vi "Gradient Read Array.vi"(8 "error in":errorcluster, 11 "Flow Gradient in":refnum<class "Flow Gradient.lvclass">) -> (0 "error out":errorcluster, 1 "Changed or First Call?":bool, 2 "Flow SP":dbl[](array[numeric]), 3 "Flow Gradient out":refnum<class "Flow Gradient.lvclass">)   [LabVIEW 2023, in "Flow Gradient.lvclass"]
uses:
  Flow Gradient.lvclass
  Parents/Gradient/Gradient.lvclass
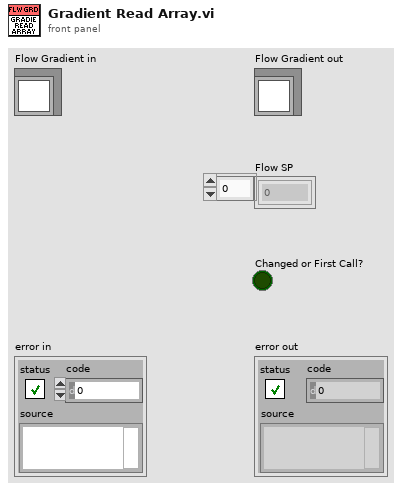
[diagram p1: front panel]
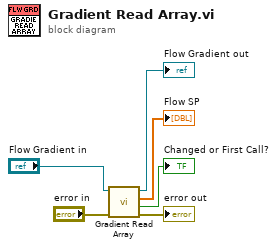
[diagram p0: block diagram]
diagram:
  n1 = call-parent "Gradient Read Array.vi"("error in"="error in", "Gradient in"="Flow Gradient in") -> ("error out"=→"error out":errorcluster, "Changed or First Call?"=→"Changed or First Call?":bool, "Current SP"=→"Flow SP":dbl[], "Gradient out"=→"Flow Gradient out":refnum<class "Flow Gradient.lvclass">)  [unwired: 6 in]
